vi "calculate_extinction_center_xi_non_zero.vi"(8 "Error In":errorcluster, 11 "Xtal Description":T1) -> (0 "Error Out":errorcluster, 3 "prediction":dbl)   [LabVIEW 2019]
uses:
  xtal_description_for_prediction_cluster_typedef.ctl
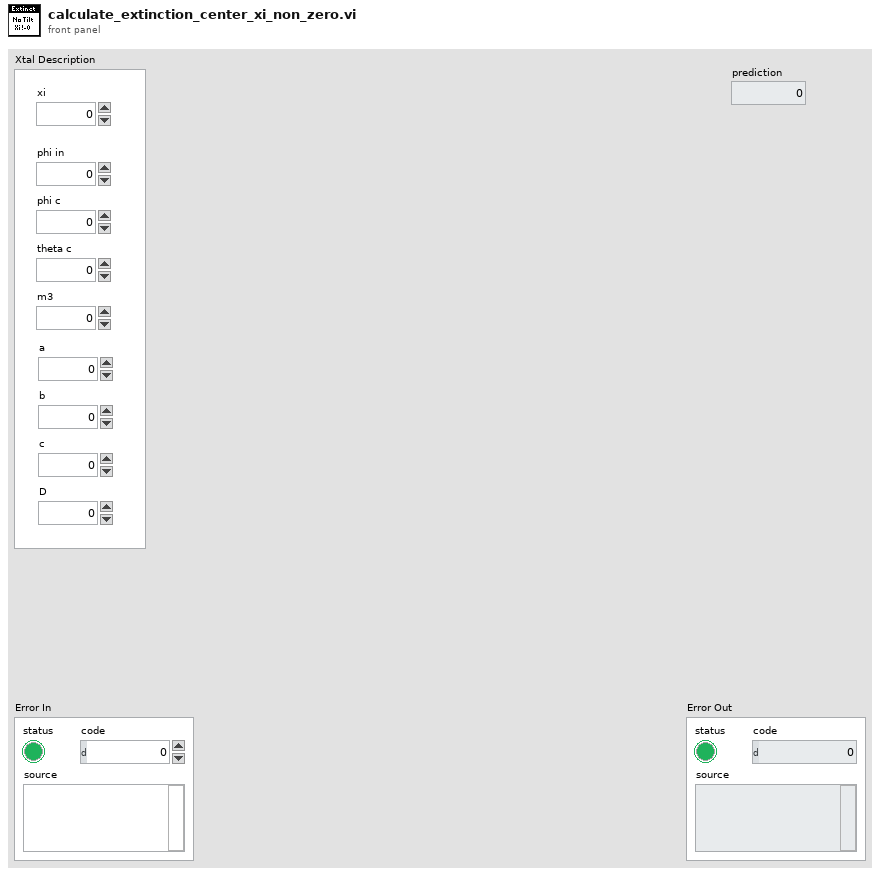
[diagram p1: front panel]
types:
  T1 = typedef "xtal_description_for_prediction_cluster_typedef.ctl" = cluster{"xi":dbl, "phi in":dbl, "phi c":dbl, "theta c":dbl, "m3":dbl, "a":dbl, "b":dbl, "c":dbl, "D":dbl}
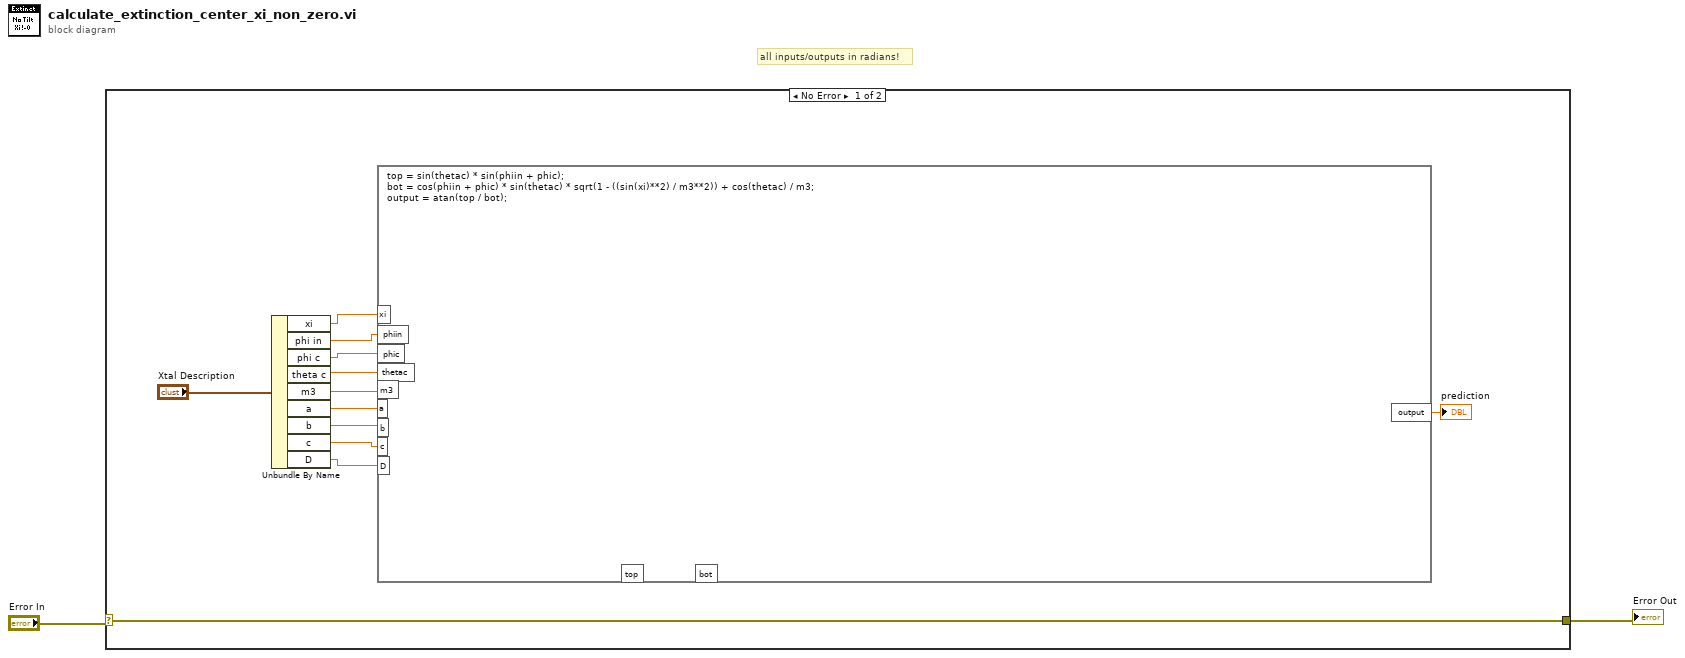
[diagram p0: block diagram]
diagram:
  # "all inputs/outputs in radians!"
  n1 = case shown="No Error" "Error In" {
    selector: "Error In" -> [w3 w15]
    tunnel: [w3 w15] -> w1
    frame No Error {
      n2 = Unbundle By Name("Xtal Description") -> ("xi"=w13:dbl, "phi in"=w12:dbl, "phi c"=w11:dbl, "theta c"=w10:dbl, "m3"=w9:dbl, "a"=w8:dbl, "b"=w7:dbl, "c"=w6:dbl, "D"=w5:dbl)
      n3 = formula code="top = sin(thetac) * sin(phiin + phic);\nbot = cos(phiin + phic) * sin(thetac) * sqrt(1 - ((sin(xi)**2) / m3**2)) + cos(thetac) / m3;\noutput = atan(top / bot);"("xi"=w13, "phiin"=w12, "phic"=w11, "thetac"=w10, "m3"=w9, "a"=w8, "b"=w7, "c"=w6, "D"=w5) -> ("output"=→"prediction":dbl)  [unwired: 2 out]
    }
    frame Error {
    }
  }
  "Error Out" <- w1
